vi "Set_Reference_Reference_Array.vi"(8 "error in (no error)":errorcluster, 10 "Reference_Reference_Array":refnum<k20>[](array[refnum]), 11 "SoftmotionAxis in":refnum<class "SoftmotionAxis.lvclass">) -> (0 "error out":errorcluster, 3 "SoftmotionAxis out":refnum<class "SoftmotionAxis.lvclass">)   [LabVIEW 2017, in "SoftmotionAxis.lvclass"]
uses:
  SoftmotionAxis.lvclass
  SoftmotionAxis.lvclass/SoftmotionAxis.ctl
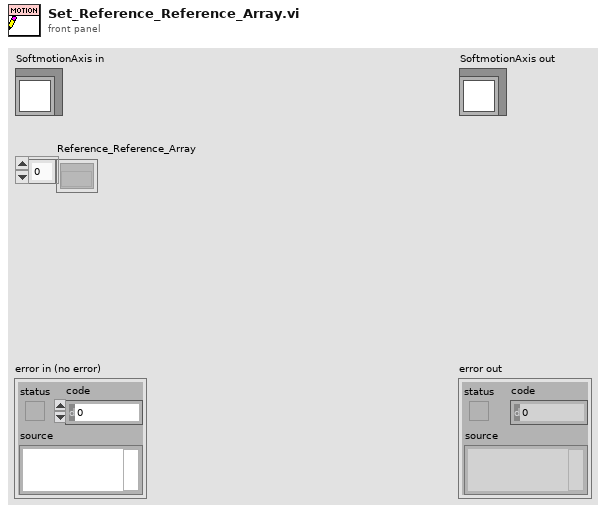
[diagram p1: front panel]
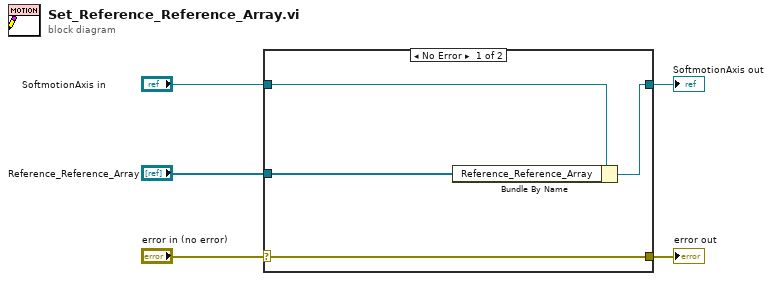
[diagram p0: block diagram]
diagram:
  n1 = case shown="No Error" "error in (no error)" {
    selector: "error in (no error)" -> [w9 w10]
    tunnel: [w9 w10] -> w4
    tunnel: [w7 w11] -> w2
    tunnel: "SoftmotionAxis in" -> [w8 w11]
    tunnel: "Reference_Reference_Array" -> [w6 _]
    frame No Error {
      n2 = Bundle By Name(cluster=w8, "Reference_Reference_Array"=w6) -> (w7:refnum<class "SoftmotionAxis.lvclass">)
    }
    frame Error {
    }
  }
  "error out" <- w4
  "SoftmotionAxis out" <- w2
